vi "Create Transfer Group Timing.vi"(7 "id":i32, 8 "error in (no error)":errorcluster, 10 "Return FIFO":refnum<k33>, 11 "cycle timing":T1) -> (0 "error out":errorcluster, 3 "Transfer Group Timing out":refnum<class "Transfer Group Timing.lvclass">)   [LabVIEW 2017, in "DSF Core.lvlib" / "Transfer Group Timing.lvclass"]
uses:
  Transfer Group Timing.lvclass
  C:/Git/DSF/Data Sharing Framework/Source/Core/Engine/Classes/Timing/Timing.lvclass
  DSF Configuration API/Public/Controls/DSF Timing Info.ctl
  Transfer Group Timing.lvclass/Transfer Group Timing.ctl
  Timing.lvclass
  DSF Core.lvlib
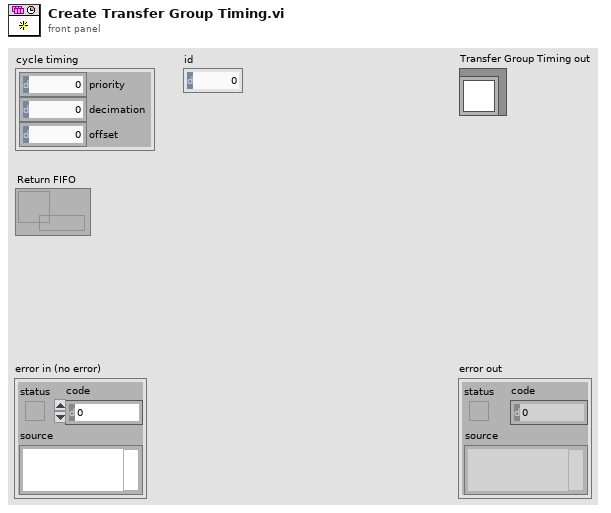
[diagram p1: front panel]
types:
  T1 = typedef "DSF Core.lvlib/DSF Timing Info.ctl" = cluster{"priority":u64, "decimation":u64, "offset":u64}
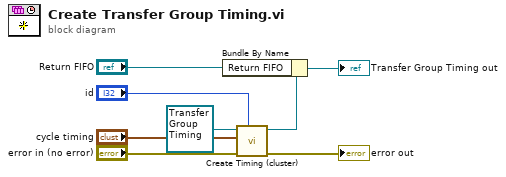
[diagram p0: block diagram]
diagram:
  n1 = call "Create Timing (cluster).vi"("id (0)"="id", "error in (no error)"="error in (no error)", "cycle timing"="cycle timing", "Timing in"=refnum<class "Transfer Group Timing.lvclass"> refnum ("Transfer Group Timing in")) -> ("error out"=→"error out":errorcluster, "Timing"=w4:refnum<class "Transfer Group Timing.lvclass">)  [unwired: 6 in]
  n2 = Bundle By Name(cluster=w4, "Return FIFO"="Return FIFO") -> (→"Transfer Group Timing out":refnum<class "Transfer Group Timing.lvclass">)
